vi "cmamo.vi"() -> ()   [LabVIEW 2015]
panel:
  in  "stop":bool
  in  "Consumo Litros/Segundo":dbl(slide) scale=0.0..1.0
  out "Grafico nivel de agua sobre tiempo":dbl(graph)
  out "Tank":dbl(slide) scale=0.0..200.0
  out "NIVEL":dbl
  out "Multi-Segment Pipe":bool(c317)
  in  "Nivel Bajo":dbl
  in  "Nivel Alto":dbl
  in  "Bomba":bool
  out "Boolean 2":bool
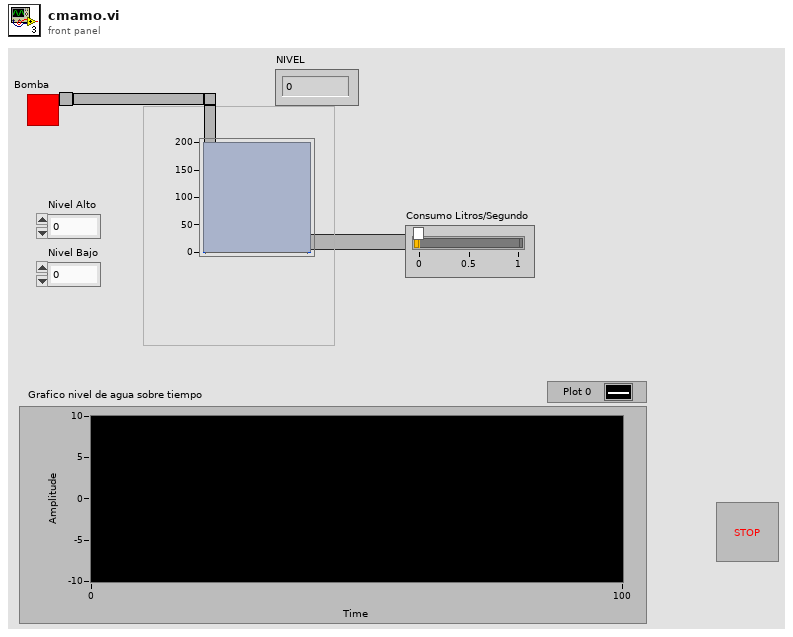
[diagram p1: front panel]
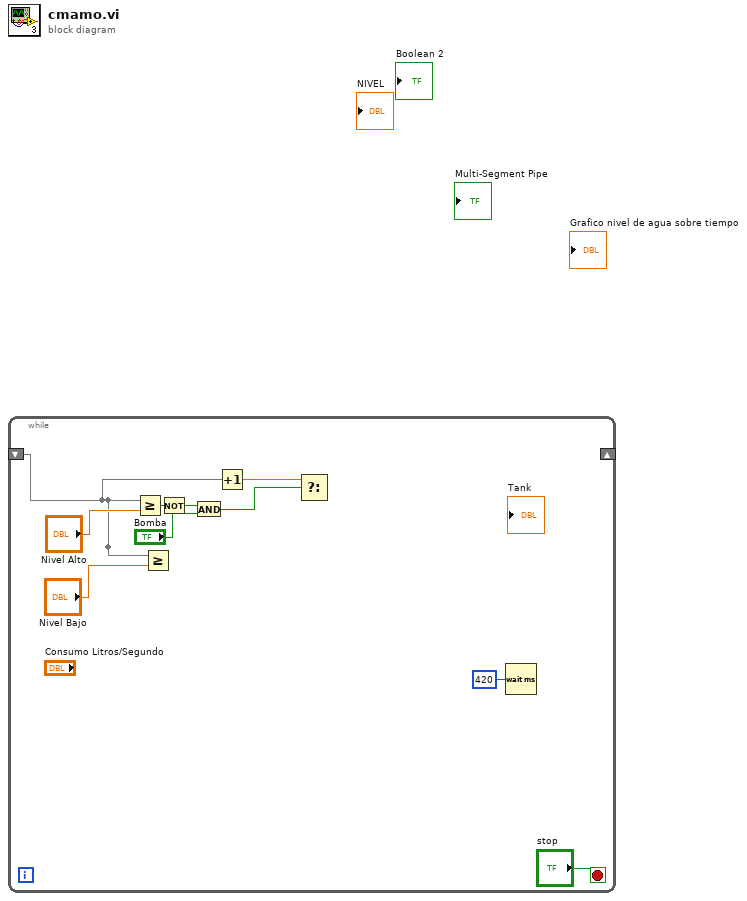
[diagram p0: block diagram]
diagram:
  n1 = while {
    shift-right: _ -> [_]
    shift-left: _ -> [w1]
    stop <- "stop" stop-if-true
    n2 = Greater Or Equal?(x=w1, y="Nivel Alto") -> (x >= y?=w4:bool)
    n3 = Greater Or Equal?(x=w1, y="Nivel Bajo") -> ()  [unwired: 1 out]
    n4 = Not(x=w4) -> (.not. x?=w5:bool)
    n5 = And(x=w5, y="Bomba") -> (x .and. y?=w3:bool)
    n6 = Increment(x=w1) -> (x+1=w2:dbl)
    n7 = Select(t=w2, s=w3) -> ()  [unwired: 1 in, 1 out]
    n8 = Wait (ms)(milliseconds to wait=u32 420) -> ()  [unwired: 1 out]
  }
